vi "Add to Tree (Internal).vi"(6 "Display Text Override":string, 7 "Add children? (F)":bool, 8 "error in (no error)":errorcluster, 9 "Parent Tag":string, 10 "Tree Manager in":refnum<class "Tree Manager.lvclass">, 11 "Data Item in":refnum<class "Data Item.lvclass">) -> (0 "error out":errorcluster, 1 "New Tag":string, 2 "Tree Manager out":refnum<class "Tree Manager.lvclass">, 3 "Data Item out":refnum<class "Data Item.lvclass">)   [LabVIEW 2018, in "VILab.lvlib" / "Data Item.lvclass"]
uses:
  Data Item.lvclass
  Tree Manager.lvclass
  Data Item.lvclass/Data Item.ctl
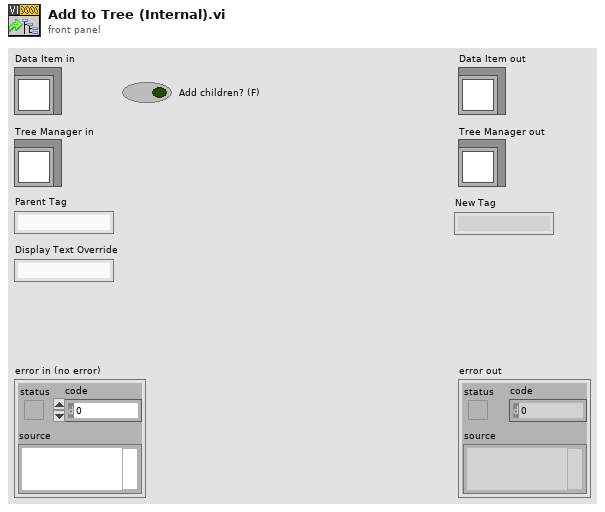
[diagram p1: front panel]
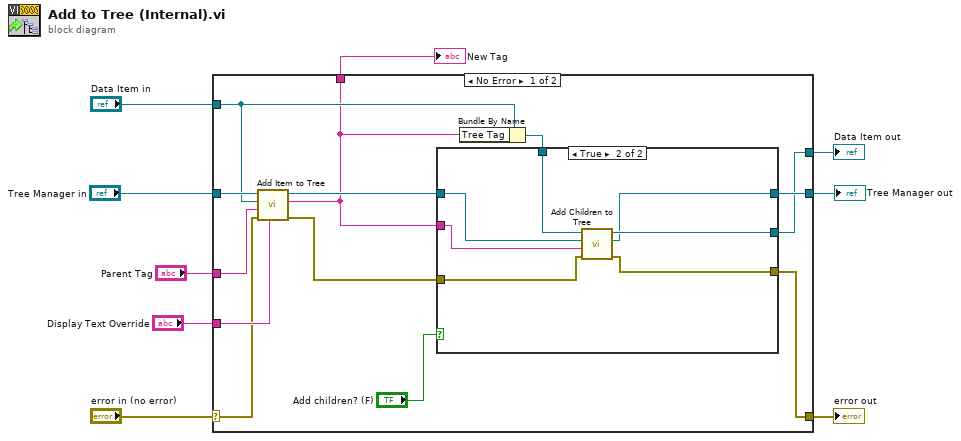
[diagram p0: block diagram]
diagram:
  n1 = case shown="No Error" "error in (no error)" {
    selector: "error in (no error)" -> [w11 w35]
    tunnel: [w15 w35] -> w8
    tunnel: [w16 w34] -> w6
    tunnel: "Data Item in" -> [w12 w34]
    tunnel: "Tree Manager in" -> [w22 w33]
    tunnel: "Parent Tag" -> [w21 _]
    tunnel: [w18 w33] -> w3
    tunnel: "Display Text Override" -> [w13 _]
    tunnel: [w10 _] -> w1
    frame No Error {
      n2 = call "Add Item to Tree.vi"("Display Text Override"=w13, "error in (no error)"=w11, "Parent Tag"=w21, "Data Item"=w12, "Tree Manager in"=w22) -> ("error out"=w19:errorcluster, "New Tag"=w10:string, "Tree Manager out"=w20:refnum<class "Tree Manager.lvclass">)  [unwired: 4 in]
      n3 = Bundle By Name(cluster=w12, "Tree Tag"=w10) -> (w17:refnum<class "Data Item.lvclass">)
      n4 = case shown="True" "Add children? (F)" {
        tunnel: w20 -> [w24 w32]
        tunnel: w19 -> [w23 w30]
        tunnel: w10 -> [_ w31]
        tunnel: [w24 w28] -> w18
        tunnel: w17 -> [w25 w26]
        tunnel: [w25 w29] -> w16
        tunnel: [w23 w27] -> w15
        frame False {
        }
        frame True {
          n5 = call "Add Children to Tree.vi"("error in (no error)"=w30, "Parent Tag"=w31, "Tree Manager in"=w32, "Data Item in"=w26) -> ("error out"=w27:errorcluster, "Tree Manager out"=w28:refnum<class "Tree Manager.lvclass">, "Data Item out"=w29:refnum<class "Data Item.lvclass">)  [unwired: 5 in]
        }
      }
    }
    frame Error {
    }
  }
  "error out" <- w8
  "Data Item out" <- w6
  "Tree Manager out" <- w3
  "New Tag" <- w1
